vi "FiberMRI_Main_Protocol_NI.vi"() -> ()   [LabVIEW 2011]
doc: "Acquisition software for combined single-photon fluorescence and fMRI experiments."
uses:
  typedefs/storage_parameters_cluster.ctl
  typedefs/protocol_parameters.ctl
  typedefs/device_parameters.ctl
  typedefs/free_run_parameters.ctl
  typedefs/run_mode.ctl
  typedefs/main_state_enum.ctl
  typedefs/control_daq_enum.ctl
  typedefs/control_display_enum.ctl
  typedefs/control_storage_enum.ctl
  typedefs/control_analysis_enum.ctl
  <vilib>/Utility/error.llb/DialogType.ctl
  typedefs/control_shutter_enum.ctl
  typedefs/control_stim_enum.ctl
  typedefs/all_frontpanel_parameters_protocol_NI.ctl
  typedefs/experiment_mode_enum.ctl
  globals/exit.vi
panel:
  in  "Run mode":T1
  in  "Tab Control":T2(tab)
  in  "Protocol parameters":T3={"Repetitions"=1.0, "ON time"=40.0, "OFF time"=120.0, "Stim onset"=5.0, "Stim frequency"=1.0, "Pulse width"=1.0, "Acquire before ON"=1.0, "Acquire after ON"=1.0, "Sync shutter to acquisition"=TRUE} {"Pulse width" min=0.0001 max=0.1 step=0.01; "Acquire after ON" min=0.0 max=20.0 step=1.0; "Acquire before ON" min=0.0 max=20.0 step=1.0; "Repetitions" min=1.0 max=10.0 step=1.0; "OFF time" min=0.0 max=1000.0; "ON time" min=0.0 max=1000.0; "Stim onset" min=0.0 max=6000.0; "Stim frequency" min=-2.0 max=40.0 step=1.0}
  in  "Free run parameters":T4={"Stim onset"=5.0, "Stim frequency"=1.0, "Stim length"=0.001, "Sync shutter to acquisition"=TRUE} {"Stim length" min=0.0001 max=0.1 step=0.01; "Stim onset" min=0.0 max=100.0; "Stim frequency" min=0.1 max=40.0 step=1.0}
  in  "Storage parameters":T5
  in  "Device parameters":T6={"Triggered?"=FALSE, "Shutter channel"="", "Acquisition channels"="", "Acquisition sample rate"=100.0, "Read chunk size"=0, "Stimulation channel"="Dev1/ao0", "Stimulation sample rate"=100.0} {"Read chunk size" min=100 max=100000; "Acquisition sample rate" min=10.0 max=10000.0 step=10.0; "Stimulation sample rate" min=10.0 max=10000.0}
  out "Running":bool
  in  "Shutter":bool
  in  "Run":bool
  in  "Quit":bool
  # "Fiber - fMRI"
  # "_0000.txt"
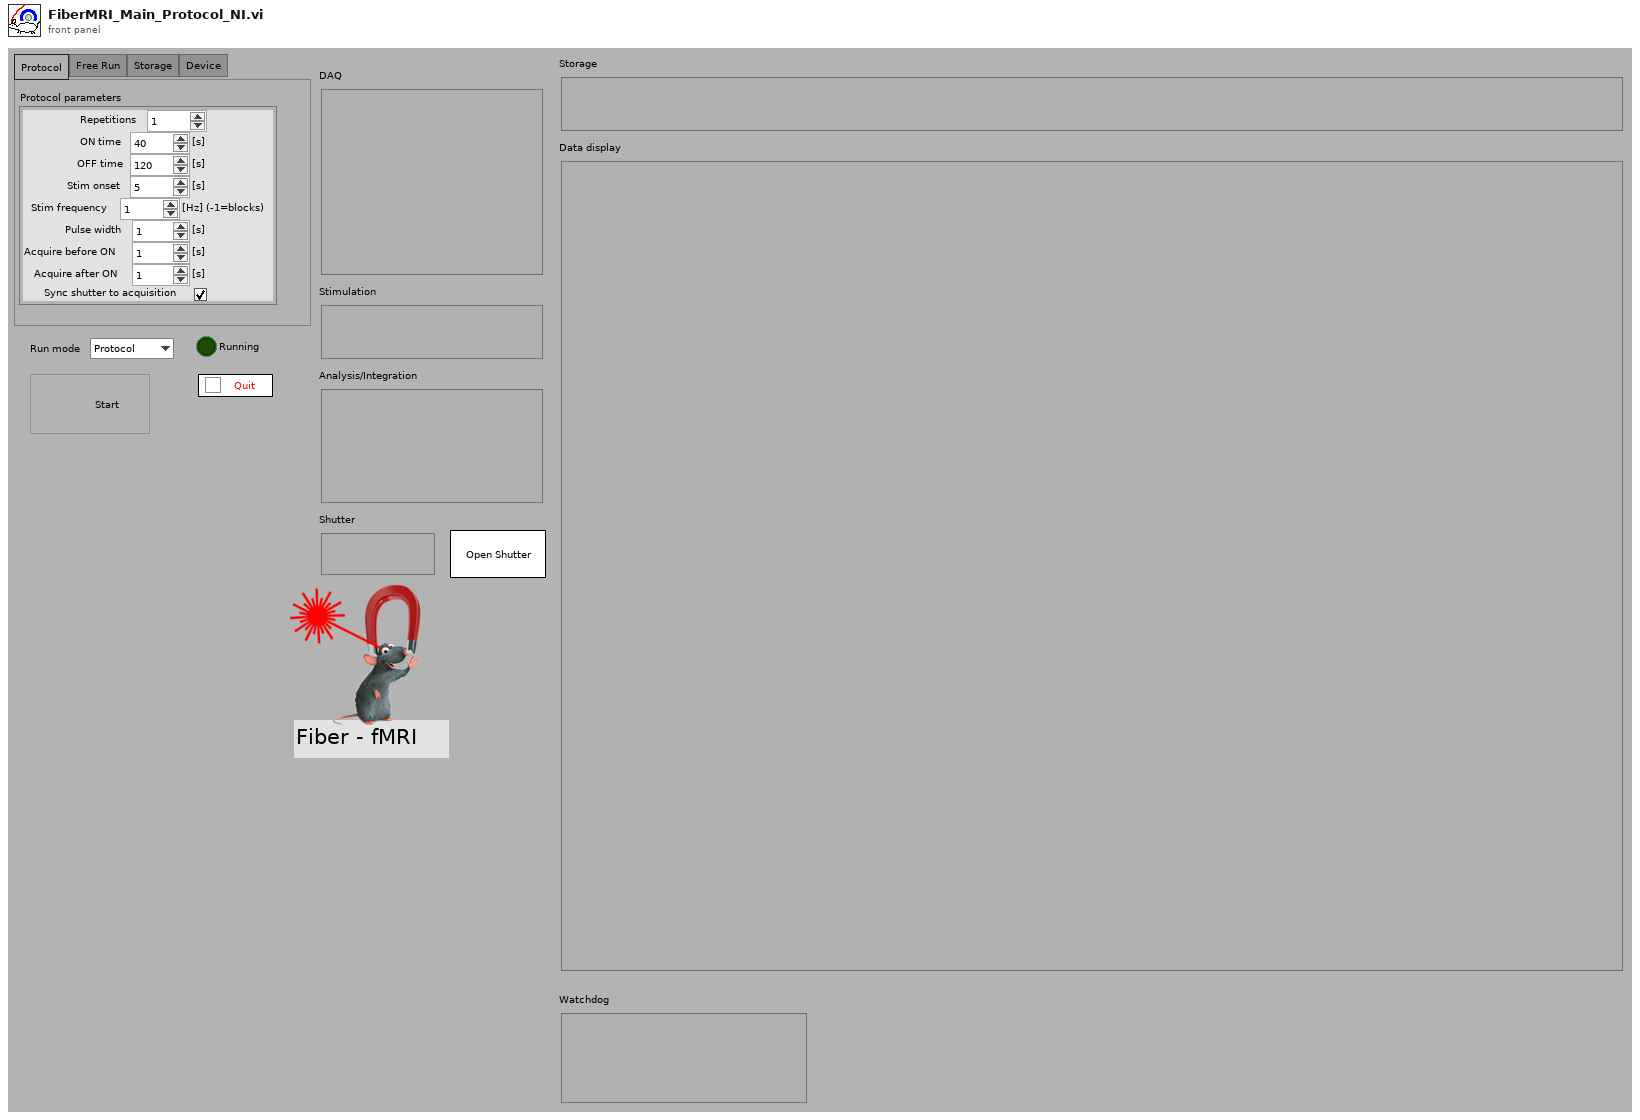
[diagram p1: front panel]
types:
  T1 = typedef "run_mode.ctl" = enum32{"Protocol", "Free Run"}
  T2 = enum32{"Protocol", "Free Run", "Storage", "Device"}
  T3 = typedef "protocol_parameters.ctl" = cluster{"Repetitions":dbl, "ON time":dbl, "OFF time":dbl, "Stim onset":dbl, "Stim frequency":dbl, "Pulse width":dbl, "Acquire before ON":dbl, "Acquire after ON":dbl, "Sync shutter to acquisition":bool}
  T4 = typedef "free_run_parameters.ctl" = cluster{"Stim onset":dbl, "Stim frequency":dbl, "Stim length":dbl, "Sync shutter to acquisition":bool}
  T5 = typedef "storage_parameters_cluster.ctl" = cluster{"Store?":bool, "Path":path, "Basename":string, "Auto-increment?":bool}
  T6 = typedef "device_parameters.ctl" = cluster{"Triggered?":bool, "Shutter channel":tag, "Acquisition channels":tag, "Acquisition sample rate":dbl, "Read chunk size":i32, "Stimulation channel":tag, "Stimulation sample rate":dbl}
  T7 = typedef "all_frontpanel_parameters_protocol_NI.ctl" = cluster{"Run mode":T1, "Protocol parameters":T3, "Free run parameters":T4, "Device parameters":T6, "Storage parameters":T5}
  T8 = typedef "DialogType.ctl" = u16
  T9 = typedef "main_state_enum.ctl" = enum16{"Init", "Empty", "ParamsChanged", "Start", "Stop", "Abort", "Acquisition finished", "SetShutter", "Reset", "Error", "Quit"}
  T10 = cluster{"Control_Stim_Queue":refnum<queue>, "Control_DAQ_Queue":refnum<queue>, "Control_Storage_Queue":refnum<queue>, "Control_Display_Queue":refnum<queue>, "Control_Analysis_Queue":refnum<queue>, "Control_Shutter_Queue":refnum<queue>}
  T11 = cluster{"Run mode":refnum<vi>, "Run":refnum<vi>, "Protocol parameters":refnum<vi>, "Tab Control":refnum<vi>, "Free run parameters":refnum<vi>, "Device parameters":refnum<vi>, "Storage parameters":refnum<vi>, "Shutter":refnum<vi>, "Quit":refnum<vi>}
  T12 = typedef "control_stim_enum.ctl" = enum16{"Init", "Stim Protocol", "Stim Free Run", "Stop", "Quit"}
  T13 = cluster{"Control stim Enum":T12, "variant":variant}
  T14 = typedef "control_shutter_enum.ctl" = enum16{"Init", "Open", "Close", "Quit"}
  T15 = cluster{"Control shutter enum":T14, "variant":variant}
  T16 = typedef "control_analysis_enum.ctl" = enum16{"Init", "Analyze", "Reset", "Stop", "Quit"}
  T17 = cluster{"Control Analysis Enum":T16, "variant":variant}
  T18 = typedef "control_display_enum.ctl" = enum16{"Init", "Display", "Quit"}
  T19 = cluster{"Control display enum":T18, "variant":variant}
  T20 = typedef "control_storage_enum.ctl" = enum16{"Init", "Discard", "Store", "Reset", "Stop", "Quit"}
  T21 = cluster{"Control storage enum":T20, "variant":variant}
  T22 = typedef "control_daq_enum.ctl" = enum16{"Init", "FreeRun", "Protocol", "Stop", "Quit"}
  T23 = cluster{"Control DAQ Enum":T22, "variant":variant}
  T24 = typedef "experiment_mode_enum.ctl" = enum32{"Raw data", "Measure background", "Measure F0", "Measure DF/F"}
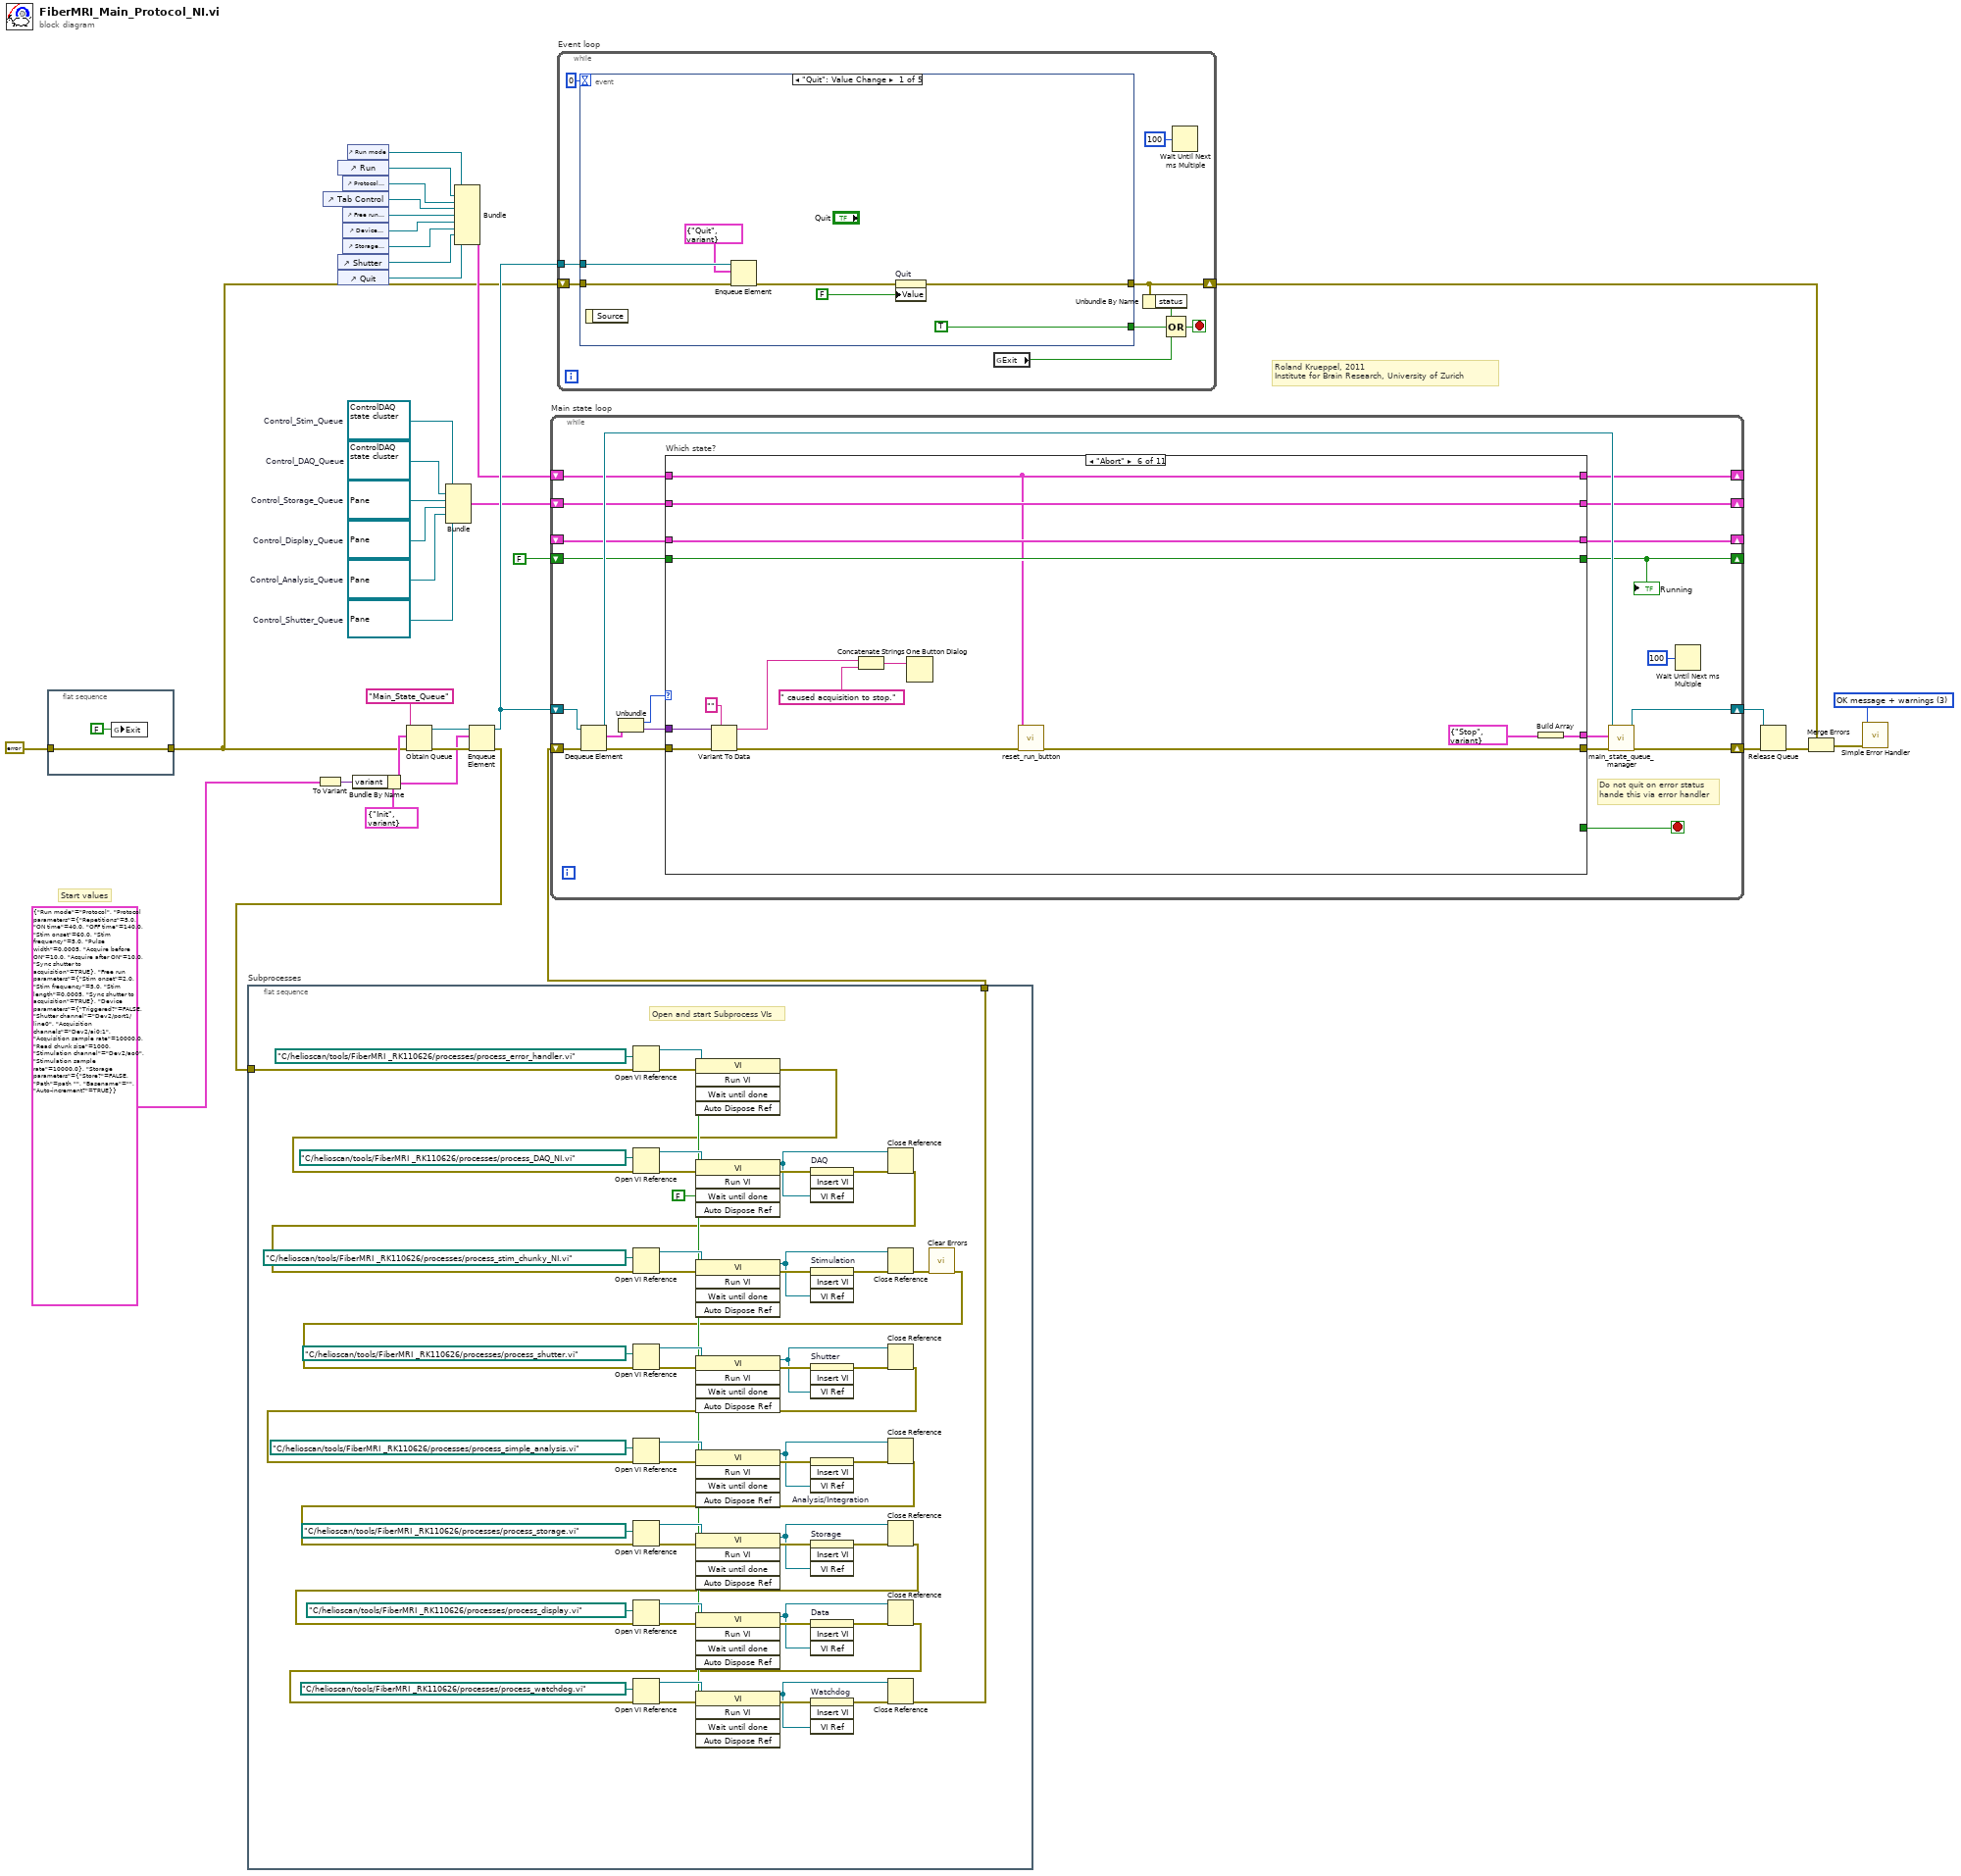
[diagram p0: block diagram]
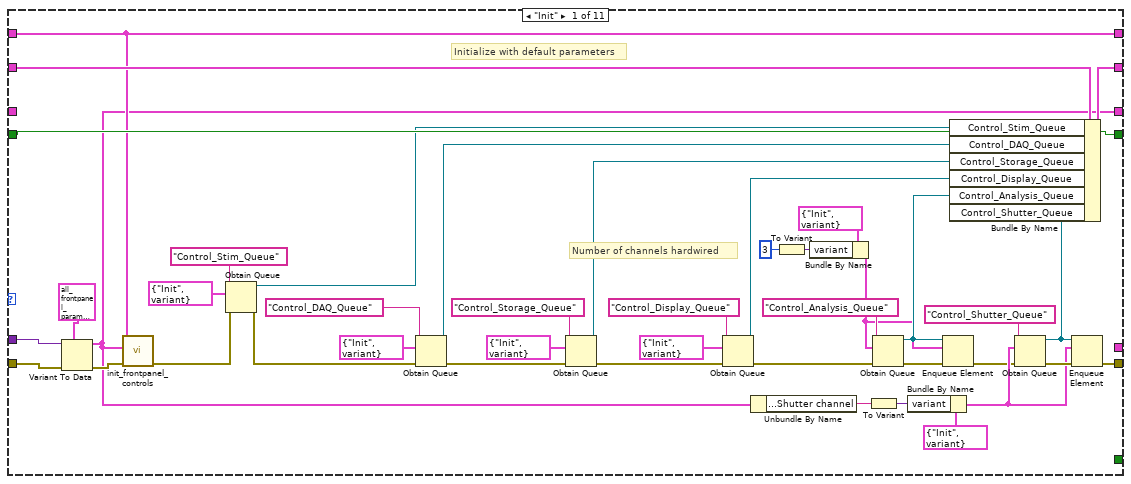
[diagram p2: hidden frame]
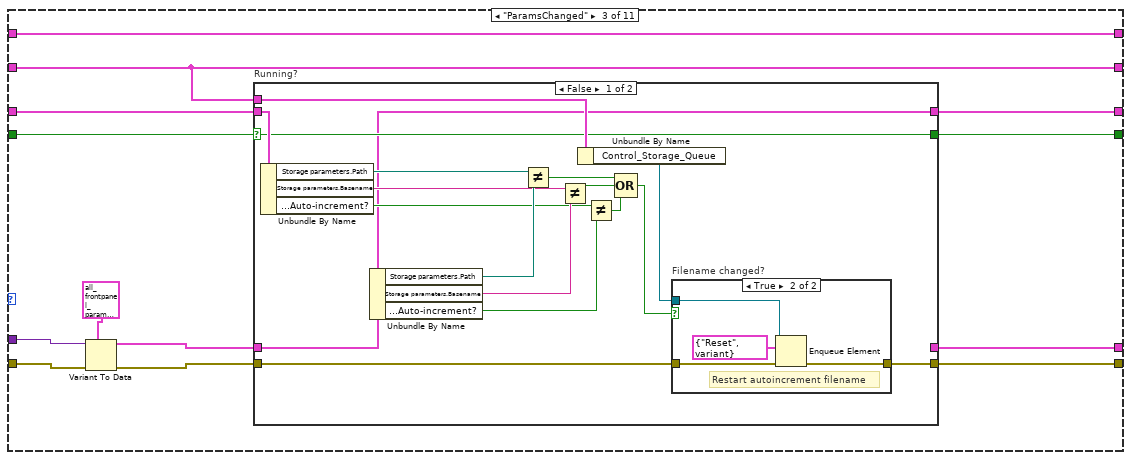
[diagram p4: hidden frame]
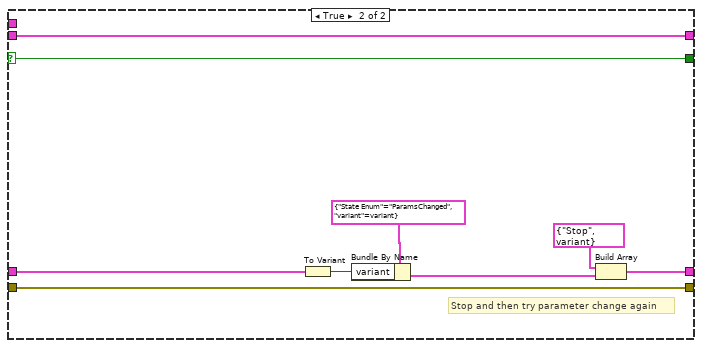
[diagram p6: hidden frame]
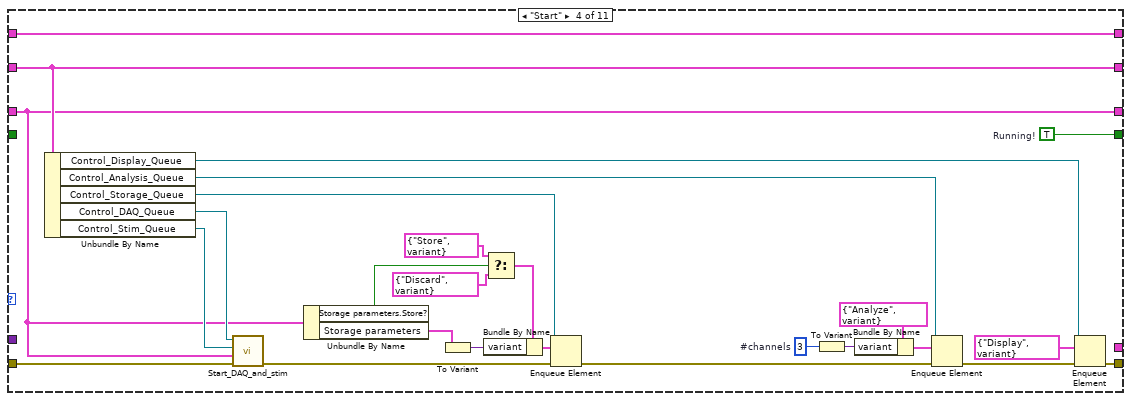
[diagram p7: hidden frame]
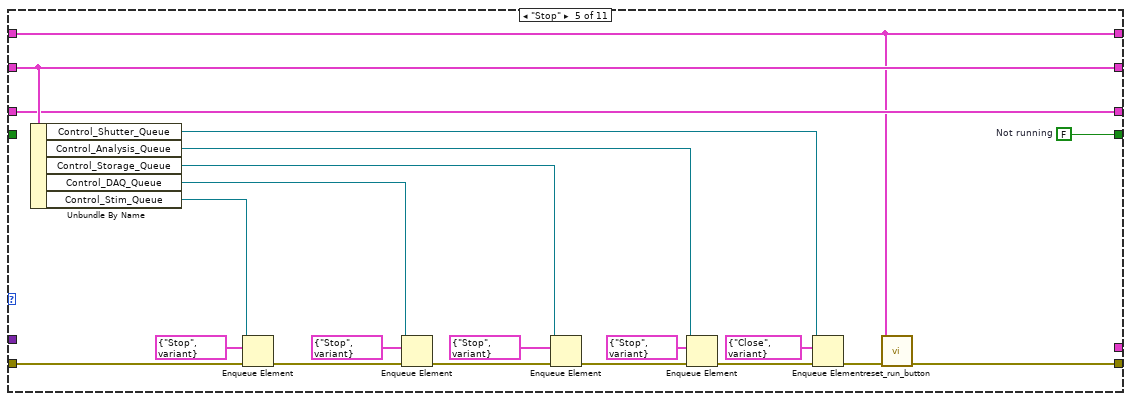
[diagram p8: hidden frame]
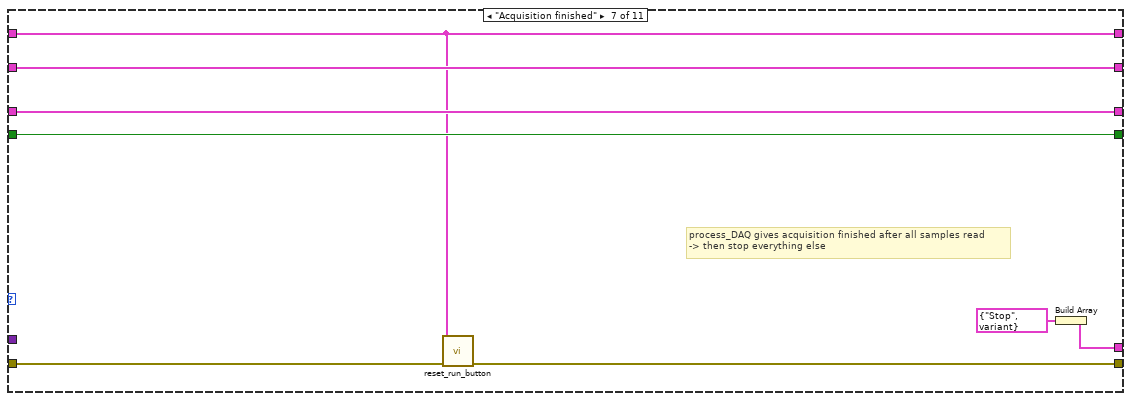
[diagram p9: hidden frame]
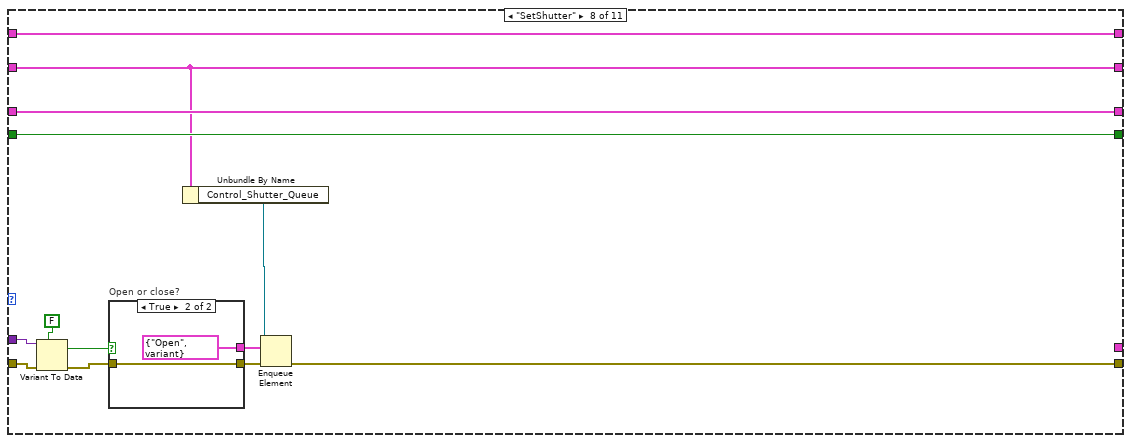
[diagram p10: hidden frame]
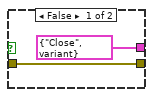
[diagram p11: hidden frame]
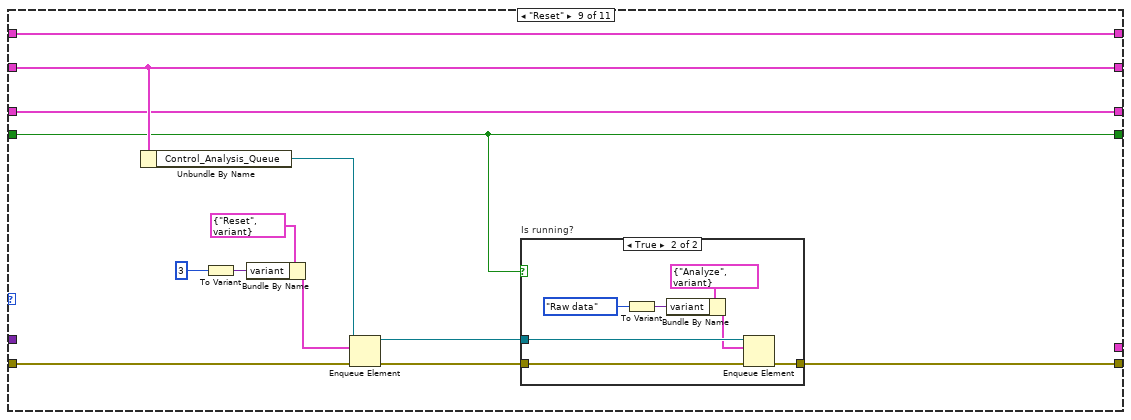
[diagram p12: hidden frame]
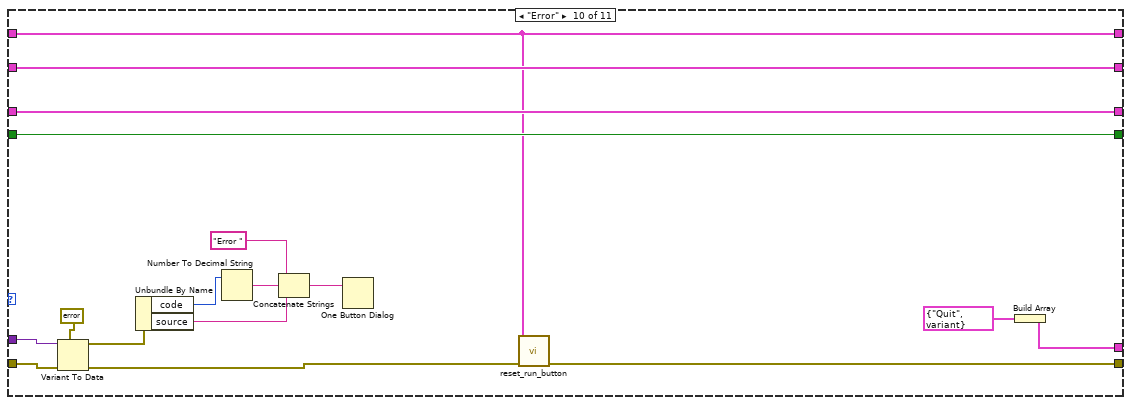
[diagram p14: hidden frame]
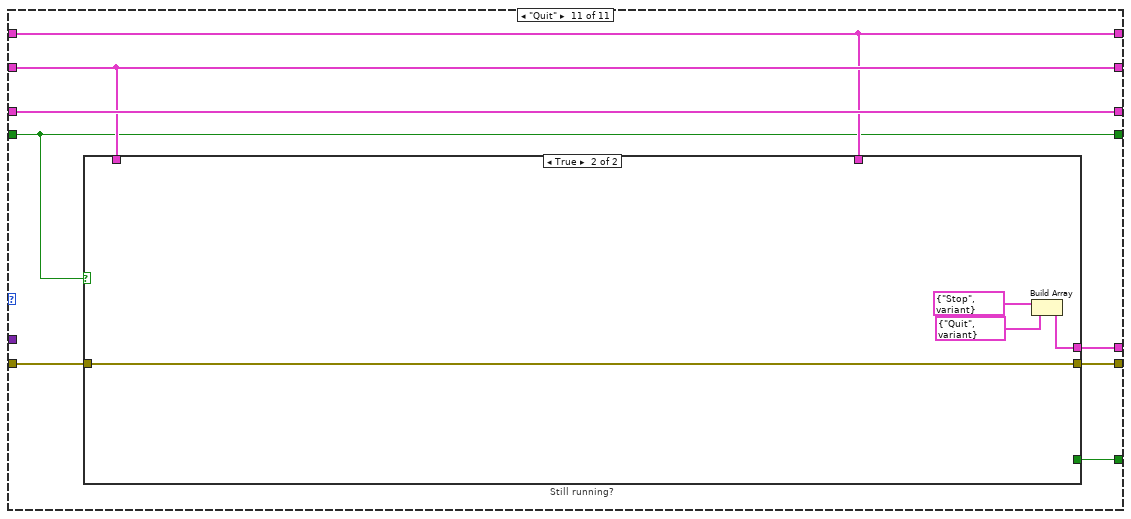
[diagram p15: hidden frame]
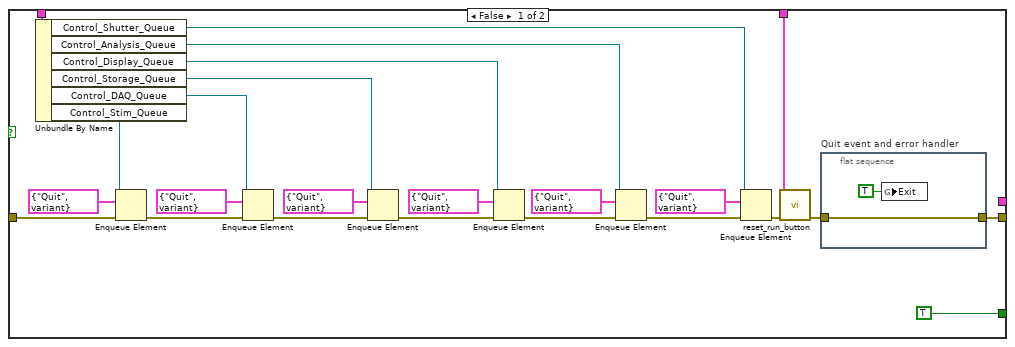
[diagram p16: hidden frame]
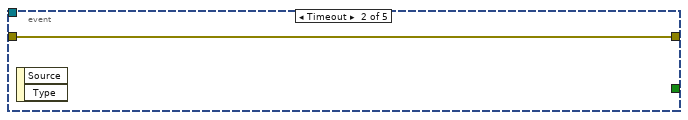
[diagram p17: hidden frame]
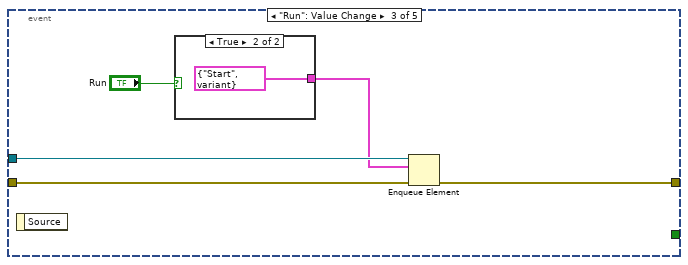
[diagram p18: hidden frame]
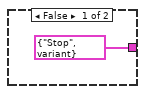
[diagram p19: hidden frame]
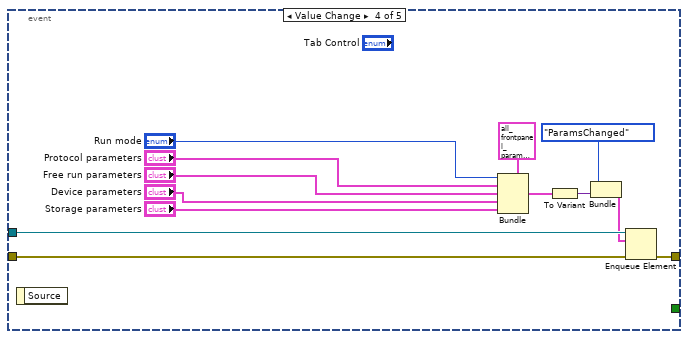
[diagram p20: hidden frame]
diagram:
  w16 = refnum<queue> refnum  # Control_Stim_Queue
  w17 = refnum<queue> refnum  # Control_Shutter_Queue
  w25 = T8 3 items=["no dialog", "OK message", "continue or stop message", "OK message + warnings", "continue/stop + warnings"] ("type of dialog (OK msg:1)")
  w26 = refnum<queue> refnum  # Control_Analysis_Queue
  w27 = refnum<queue> refnum  # Control_Storage_Queue
  w28 = refnum<queue> refnum  # Control_Display_Queue
  w30 = refnum<queue> refnum  # Control_DAQ_Queue
  # "Start values"
  # "Roland Krueppel, 2011\nInstitute for Brain Research, University of Zurich"
  n1 = flat-sequence {
    tunnel: errorcluster {"status"=FALSE, "code"=0, "source"=""} ("error out") -> [w37]
    tunnel: [w37] -> w3
    frame #0 {
      n2 = global write "exit.vi" "Exit"(FALSE ("Exit")) -> ()
    }
  }
  n3 = flat-sequence "Subprocesses" {
    tunnel: w2 -> [w43]
    tunnel: [w41] -> w1
    frame #0 {
      w49 = FALSE ("Wait Until Done")
      # "Open and start Subprocess VIs"
      n4 = Open VI Reference(vi path=path "C:/helioscan/tools/FiberMRI _RK110626/processes/process_error_handler.vi", error in (no error)=w43) -> (vi reference=w50:refnum<vi>, error out=w51:errorcluster)  [unwired: 4 in]
      n5 = invoke class="VI" method="Run VI"(reference=w50, error in=w51, "Wait until done"=w49) -> (error out=w42:errorcluster)  [unwired: 2 in, 4 out]
      n6 = Open VI Reference(vi path=path "C:/helioscan/tools/FiberMRI _RK110626/processes/process_DAQ_NI.vi", error in (no error)=w42) -> (vi reference=w89:refnum<vi>, error out=w90:errorcluster)  [unwired: 4 in]
      n7 = invoke class="VI" method="Run VI"(reference=w89, error in=w90, "Wait until done"=w49) -> (reference out=w68:refnum<vi>, error out=w70:errorcluster)  [unwired: 2 in, 3 out]
      n8 = invoke on="DAQ" class="SubPanel" method="Insert VI"(error in=w70, "VI Ref"=w68) -> (error out=w69:errorcluster)  [unwired: 2 in, 3 out]
      n9 = Close Reference(reference=w68, error in (no error)=w69) -> (error out=w48:errorcluster)
      n10 = Open VI Reference(vi path=path "C:/helioscan/tools/FiberMRI _RK110626/processes/process_stim_chunky_NI.vi", error in (no error)=w48) -> (vi reference=w58:refnum<vi>, error out=w59:errorcluster)  [unwired: 4 in]
      n11 = invoke class="VI" method="Run VI"(reference=w58, error in=w59, "Wait until done"=w49) -> (reference out=w54:refnum<vi>, error out=w56:errorcluster)  [unwired: 2 in, 3 out]
      n12 = invoke on="Stimulation" class="SubPanel" method="Insert VI"(error in=w56, "VI Ref"=w54) -> (error out=w55:errorcluster)  [unwired: 2 in, 3 out]
      n13 = Close Reference(reference=w54, error in (no error)=w55) -> (error out=w40:errorcluster)
      n14 = call <vilib>:"Clear Errors.vi"("error in (no error)"=w40) -> ("error out"=w39:errorcluster)  [unwired: 6 in]
      n15 = Open VI Reference(vi path=path "C:/helioscan/tools/FiberMRI _RK110626/processes/process_shutter.vi", error in (no error)=w39) -> (vi reference=w53:refnum<vi>, error out=w63:errorcluster)  [unwired: 4 in]
      n16 = invoke class="VI" method="Run VI"(reference=w53, error in=w63, "Wait until done"=w49) -> (reference out=w60:refnum<vi>, error out=w62:errorcluster)  [unwired: 2 in, 3 out]
      n17 = invoke on="Shutter" class="SubPanel" method="Insert VI"(error in=w62, "VI Ref"=w60) -> (error out=w61:errorcluster)  [unwired: 2 in, 3 out]
      n18 = Close Reference(reference=w60, error in (no error)=w61) -> (error out=w47:errorcluster)
      n19 = Open VI Reference(vi path=path "C:/helioscan/tools/FiberMRI _RK110626/processes/process_simple_analysis.vi", error in (no error)=w47) -> (vi reference=w87:refnum<vi>, error out=w88:errorcluster)  [unwired: 4 in]
      n20 = invoke class="VI" method="Run VI"(reference=w87, error in=w88, "Wait until done"=w49) -> (reference out=w79:refnum<vi>, error out=w82:errorcluster)  [unwired: 2 in, 3 out]
      n21 = invoke on="Analysis/Integration" class="SubPanel" method="Insert VI"(error in=w82, "VI Ref"=w79) -> (error out=w80:errorcluster)  [unwired: 2 in, 3 out]
      n22 = Close Reference(reference=w79, error in (no error)=w80) -> (error out=w46:errorcluster)
      n23 = Open VI Reference(vi path=path "C:/helioscan/tools/FiberMRI _RK110626/processes/process_storage.vi", error in (no error)=w46) -> (vi reference=w85:refnum<vi>, error out=w86:errorcluster)  [unwired: 4 in]
      n24 = invoke class="VI" method="Run VI"(reference=w85, error in=w86, "Wait until done"=w49) -> (reference out=w65:refnum<vi>, error out=w67:errorcluster)  [unwired: 2 in, 3 out]
      n25 = invoke on="Storage" class="SubPanel" method="Insert VI"(error in=w67, "VI Ref"=w65) -> (error out=w66:errorcluster)  [unwired: 2 in, 3 out]
      n26 = Close Reference(reference=w65, error in (no error)=w66) -> (error out=w45:errorcluster)
      n27 = Open VI Reference(vi path=path "C:/helioscan/tools/FiberMRI _RK110626/processes/process_display.vi", error in (no error)=w45) -> (vi reference=w83:refnum<vi>, error out=w84:errorcluster)  [unwired: 4 in]
      n28 = invoke class="VI" method="Run VI"(reference=w83, error in=w84, "Wait until done"=w49) -> (reference out=w77:refnum<vi>, error out=w81:errorcluster)  [unwired: 2 in, 3 out]
      n29 = invoke on="Data" class="SubPanel" method="Insert VI"(error in=w81, "VI Ref"=w77) -> (error out=w78:errorcluster)  [unwired: 2 in, 3 out]
      n30 = Close Reference(reference=w77, error in (no error)=w78) -> (error out=w44:errorcluster)
      n31 = Open VI Reference(vi path=path "C:/helioscan/tools/FiberMRI _RK110626/processes/process_watchdog.vi", error in (no error)=w44) -> (vi reference=w74:refnum<vi>, error out=w76:errorcluster)  [unwired: 4 in]
      n32 = invoke class="VI" method="Run VI"(reference=w74, error in=w76, "Wait until done"=w49) -> (reference out=w71:refnum<vi>, error out=w73:errorcluster)  [unwired: 2 in, 3 out]
      n33 = invoke on="Watchdog" class="SubPanel" method="Insert VI"(error in=w73, "VI Ref"=w71) -> (error out=w72:errorcluster)  [unwired: 2 in, 3 out]
      n34 = Close Reference(reference=w71, error in (no error)=w72) -> (error out=w41:errorcluster)
    }
  }
  n35 = To Variant(anything=T7 {"Run mode"=enum."Protocol", "Protocol parameters"={"Repetitions"=5.0, "ON time"=40.0, "OFF time"=140.0, "Stim onset"=60.0, "Stim frequency"=5.0, "Pulse width"=0.0005, "Acquire before ON"=10.0, "Acquire after ON"=10.0, "Sync shutter to acquisition"=TRUE}, "Free run parameters"={"Stim onset"=2.0, "Stim frequency"=5.0, "Stim length"=0.0005, "Sync shutter to acquisition"=TRUE}, "Device parameters"={"Triggered?"=FALSE, "Shutter channel"="Dev2/port1/line0", "Acquisition channels"="Dev2/ai0:1", "Acquisition sample rate"=10000.0, "Read chunk size"=1000, "Stimulation channel"="Dev2/ao0", "Stimulation sample rate"=10000.0}, "Storage parameters"={"Store?"=FALSE, "Path"=path "", "Basename"="", "Auto-increment?"=TRUE}} ("All frontpanel parameters")) -> (Variant=w19:variant)
  n36 = control-ref of="Tab Control"() -> (w12:refnum<vi>)
  n37 = control-ref of="Run"() -> (w14:refnum<vi>)
  n38 = control-ref of="Shutter"() -> (w8:refnum<vi>)
  n39 = control-ref of="Quit"() -> (w7:refnum<vi>)
  n40 = control-ref of="Protocol parameters"() -> (w13:refnum<vi>)
  n41 = control-ref of="Free run parameters"() -> (w11:refnum<vi>)
  n42 = control-ref of="Device parameters"() -> (w10:refnum<vi>)
  n43 = control-ref of="Storage parameters"() -> (w9:refnum<vi>)
  n44 = control-ref of="Run mode"() -> (w15:refnum<vi>)
  n45 = Bundle By Name(cluster=cluster{"State Enum":T9, "variant":variant} {"State Enum"=enum."Init", "variant"=variant}, "variant"=w19) -> (w18:cluster{"State Enum":T9, "variant":variant})
  n46 = Obtain Queue(name (unnamed)="Main_State_Queue", element data type=w18, error in (no error)=w3) -> (queue out=w35:refnum<queue>, error out=w33:errorcluster)  [unwired: 2 in, 1 out]
  n47 = Bundle("Control_Stim_Queue"=w16, "Control_DAQ_Queue"=w30, "Control_Storage_Queue"=w27, "Control_Display_Queue"=w28, "Control_Analysis_Queue"=w26, "Control_Shutter_Queue"=w17) -> (w29:T10)  [unwired: 1 in]
  n48 = Bundle("Run mode"=w15, "Run"=w14, "Protocol parameters"=w13, "Tab Control"=w12, "Free run parameters"=w11, "Device parameters"=w10, "Storage parameters"=w9, "Shutter"=w8, "Quit"=w7) -> (w6:T11)  [unwired: 1 in]
  n49 = Enqueue Element(queue=w35, element=w18, error in (no error)=w33) -> (queue out=w34:refnum<queue>, error out=w2:errorcluster)  [unwired: 1 in, 1 out]
  n50 = while "Main state loop" {
    shift-right: [w96] -> w36
    shift-left: w1 -> [w113]
    shift-right: [w108] -> _
    shift-left: _ -> [w107]
    shift-right: [w105] -> _
    shift-left: w29 -> [w106]
    shift-right: [w103] -> _
    shift-left: FALSE -> [w104]
    shift-right: [w97] -> _
    shift-left: w6 -> [w98]
    shift-right: [w99] -> w32
    shift-left: w34 -> [w114]
    stop <- w95 stop-if-true
    # "Do not quit on error status\nhande this via error handler"
    n51 = Dequeue Element(queue=w114, error in (no error)=w113) -> (queue out=w115:refnum<queue>, element=w111:cluster{"State Enum":T9, "variant":variant}, error out=w112:errorcluster)  [unwired: 1 in, 1 out]
    n52 = Unbundle(w111) -> ("State Enum"=w110:T9, "variant"=w109:variant)
    n53 = case "Which state?" shown="\"Abort\"" w110 {
      tunnel: w112 -> [w141 w162 w174 w214 w242 w264 w270 w287 w304 w324 w336]
      tunnel: [w132 w162 w170 w230 w234 w255 w269 w277 w300 w327 w334] -> w101
      tunnel: w109 -> [w140 _ w175 _ _ w263 _ w286 _ w325 _]
      tunnel: [w116 w161 w165 w209 w244 w267 w275 w288 w302 w330 w338] -> w108
      tunnel: w107 -> [_ w161 w173 w209 w244 w267 w275 w288 w302 w330 w338]
      tunnel: w106 -> [w153 w160 w172 w232 w252 w266 w274 w283 w305 w329 w337]
      tunnel: [w152 w160 w172 w232 w252 w266 w274 w283 w305 w329 w337] -> w105
      tunnel: w104 -> [w142 w159 w168 _ _ w265 w271 w284 w298 w328 w333]
      tunnel: [w142 w159 w167 w221 w243 w265 w271 w284 w298 w328 w333] -> w103
      tunnel: [_ _ w164 _ _ w257 w272 _ _ w314 w332] -> w100
      tunnel: w98 -> [w117 w158 w163 w207 w233 w254 w268 w276 w293 w326 w335]
      tunnel: [w117 w158 w163 w207 w233 w254 w268 w276 w293 w326 w335] -> w97
      tunnel: [_ _ _ _ _ _ _ _ _ _ w331] -> w95
      frame "Init" {
        # "Number of channels hardwired"
        # "Initialize with default parameters"
        n54 = Variant To Data(error in=w141, type=T7 {"Run mode"=enum."Protocol", "Protocol parameters"={"Repetitions"=0.0, "ON time"=0.0, "OFF time"=0.0, "Stim onset"=0.0, "Stim frequency"=0.0, "Pulse width"=0.0, "Acquire before ON"=0.0, "Acquire after ON"=0.0, "Sync shutter to acquisition"=FALSE}, "Free run parameters"={"Stim onset"=0.0, "Stim frequency"=0.0, "Stim length"=0.0, "Sync shutter to acquisition"=FALSE}, "Device parameters"={"Triggered?"=FALSE, "Shutter channel"="", "Acquisition channels"="", "Acquisition sample rate"=0.0, "Read chunk size"=0, "Stimulation channel"="", "Stimulation sample rate"=0.0}, "Storage parameters"={"Store?"=FALSE, "Path"=path "", "Basename"="", "Auto-increment?"=FALSE}} ("All frontpanel parameters"), Variant=w140) -> (data=w116:T7, error out=w119:errorcluster)
        n55 = call "init_frontpanel_controls.vi"("error in"=w119, "All frontpanel parameters"=w116, "All frontpanel references"=w117) -> ("error out"=w118:errorcluster)  [unwired: 8 in]
        n56 = Obtain Queue(name (unnamed)="Control_Stim_Queue", element data type=T13 {"Control stim Enum"=enum."Init", "variant"=variant} ("ControlDAQ state cluster"), error in (no error)=w118) -> (queue out=w130:refnum<queue>, error out=w120:errorcluster)  [unwired: 2 in, 1 out]
        n57 = Obtain Queue(name (unnamed)="Control_DAQ_Queue", element data type=T23 {"Control DAQ Enum"=enum."Init", "variant"=variant} ("ControlDAQ state cluster"), error in (no error)=w120) -> (queue out=w151:refnum<queue>, error out=w149:errorcluster)  [unwired: 2 in, 1 out]
        n58 = Obtain Queue(name (unnamed)="Control_Storage_Queue", element data type=T21 {"Control storage enum"=enum."Init", "variant"=variant}, error in (no error)=w149) -> (queue out=w150:refnum<queue>, error out=w148:errorcluster)  [unwired: 2 in, 1 out]
        n59 = Obtain Queue(name (unnamed)="Control_Display_Queue", element data type=T19 {"Control display enum"=enum."Init", "variant"=variant}, error in (no error)=w148) -> (queue out=w145:refnum<queue>, error out=w144:errorcluster)  [unwired: 2 in, 1 out]
        n60 = Unbundle By Name(w116) -> ("Device parameters.Shutter channel"=w137:tag)
        n61 = To Variant(anything=3) -> (Variant=w125:variant)
        n62 = Bundle By Name(cluster=T17 {"Control Analysis Enum"=enum."Init", "variant"=variant}, "variant"=w125) -> (w121:T17)
        n63 = To Variant(anything=w137) -> (Variant=w135:variant)
        n64 = Obtain Queue(name (unnamed)="Control_Analysis_Queue", element data type=w121, error in (no error)=w144) -> (queue out=w122:refnum<queue>, error out=w124:errorcluster)  [unwired: 2 in, 1 out]
        n65 = Bundle By Name(cluster=T15 {"Control shutter enum"=enum."Init", "variant"=variant}, "variant"=w135) -> (w131:T15)
        n66 = Enqueue Element(queue=w122, element=w121, error in (no error)=w124) -> (error out=w123:errorcluster)  [unwired: 1 in, 2 out]
        n67 = Obtain Queue(name (unnamed)="Control_Shutter_Queue", element data type=w131, error in (no error)=w123) -> (queue out=w134:refnum<queue>, error out=w133:errorcluster)  [unwired: 2 in, 1 out]
        n68 = Bundle By Name(cluster=w153, "Control_Stim_Queue"=w130, "Control_DAQ_Queue"=w151, "Control_Storage_Queue"=w150, "Control_Display_Queue"=w145, "Control_Analysis_Queue"=w122, "Control_Shutter_Queue"=w134) -> (w152:T10)
        n69 = Enqueue Element(queue=w134, element=w131, error in (no error)=w133) -> (error out=w132:errorcluster)  [unwired: 1 in, 2 out]
      }
      frame "Empty", Default {
        # "Do nothing"
      }
      frame "ParamsChanged" {
        n70 = Variant To Data(error in=w174, type=T7 {"Run mode"=enum."Protocol", "Protocol parameters"={"Repetitions"=0.0, "ON time"=0.0, "OFF time"=0.0, "Stim onset"=0.0, "Stim frequency"=0.0, "Pulse width"=0.0, "Acquire before ON"=0.0, "Acquire after ON"=0.0, "Sync shutter to acquisition"=FALSE}, "Free run parameters"={"Stim onset"=0.0, "Stim frequency"=0.0, "Stim length"=0.0, "Sync shutter to acquisition"=FALSE}, "Device parameters"={"Triggered?"=FALSE, "Shutter channel"="", "Acquisition channels"="", "Acquisition sample rate"=0.0, "Read chunk size"=0, "Stimulation channel"="", "Stimulation sample rate"=0.0}, "Storage parameters"={"Store?"=FALSE, "Path"=path "", "Basename"="", "Auto-increment?"=FALSE}} ("All frontpanel parameters"), Variant=w175) -> (data=w166:T7, error out=w171:errorcluster)
        n71 = case "Running?" shown="False" w168 {
          selector: w168 -> [w177 w206]
          tunnel: w173 -> [w192 w199]
          tunnel: w172 -> [w181 _]
          tunnel: w171 -> [w179 w198]
          tunnel: [w178 w198] -> w170
          tunnel: w166 -> [w176 w205]
          tunnel: [w177 w206] -> w167
          tunnel: [w176 w199] -> w165
          tunnel: [_ w201] -> w164
          frame False {
            n72 = Unbundle By Name(w192) -> ("Storage parameters.Path"=w191:path, "Storage parameters.Basename"=w189:string, "Storage parameters.Auto-increment?"=w187:bool)
            n73 = Unbundle By Name(w176) -> ("Storage parameters.Path"=w190:path, "Storage parameters.Basename"=w188:string, "Storage parameters.Auto-increment?"=w186:bool)
            n74 = Not Equal?(x=w191, y=w190) -> (x != y?=w185:bool)
            n75 = Not Equal?(x=w189, y=w188) -> (x != y?=w184:bool)
            n76 = Unbundle By Name(w181) -> ("Control_Storage_Queue"=w180:refnum<queue>)
            n77 = Not Equal?(x=w187, y=w186) -> (x != y?=w183:bool)
            n78 = Compound Arithmetic op=OR(w185, w184, w183) -> (w182:bool)
            n79 = case "Filename changed?" shown="True" w182 {
              tunnel: w180 -> [_ w197]
              tunnel: w179 -> [w193 w195]
              tunnel: [w193 w194] -> w178
              frame False {
              }
              frame True {
                # "Restart autoincrement filename"
                n80 = Enqueue Element(queue=w197, element=T21 {"Control storage enum"=enum."Reset", "variant"=variant}, error in (no error)=w195) -> (error out=w194:errorcluster)  [unwired: 1 in, 2 out]
              }
            }
          }
          frame True {
            # "Stop and then try parameter change again"
            n81 = To Variant(anything=w205) -> (Variant=w203:variant)
            n82 = Bundle By Name(cluster=cluster{"State Enum":T9, "variant":variant} {"State Enum"=enum."ParamsChanged", "variant"=variant}, "variant"=w203) -> (w200:cluster{"State Enum":T9, "variant":variant})
            n83 = Build Array(cluster{"State Enum":T9, "variant":variant} {"State Enum"=enum."Stop", "variant"=variant}, w200) -> (w201:cluster{"State Enum":T9, "variant":variant}[])
          }
        }
      }
      frame "Start" {
        w208 = 3  # #channels
        w221 = TRUE  # Running!
        n84 = Unbundle By Name(w232) -> ("Control_Display_Queue"=w228:refnum<queue>, "Control_Analysis_Queue"=w225:refnum<queue>, "Control_Storage_Queue"=w231:refnum<queue>, "Control_DAQ_Queue"=w212:refnum<queue>, "Control_Stim_Queue"=w211:refnum<queue>)
        n85 = call "Start_DAQ_and_stim.vi"("error in"=w214, "All frontpanel parameters"=w209, "Control_Stim_Queue"=w211, "Control_DAQ_Queue"=w212) -> ("error out"=w213:errorcluster)  [unwired: 5 in]
        n86 = Unbundle By Name(w209) -> ("Storage parameters.Store?"=w210:bool, "Storage parameters"=w220:T5)
        n87 = To Variant(anything=w220) -> (Variant=w219:variant)
        n88 = Select(t=T21 {"Control storage enum"=enum."Store", "variant"=variant} ("element"), s=w210, f=T21 {"Control storage enum"=enum."Discard", "variant"=variant} ("element")) -> (s? t:f=w216:T21)
        n89 = Bundle By Name(cluster=w216, "variant"=w219) -> (w215:T21)
        n90 = Enqueue Element(queue=w231, element=w215, error in (no error)=w213) -> (error out=w227:errorcluster)  [unwired: 1 in, 2 out]
        n91 = To Variant(anything=w208) -> (Variant=w224:variant)
        n92 = Bundle By Name(cluster=T17 {"Control Analysis Enum"=enum."Analyze", "variant"=variant} ("element"), "variant"=w224) -> (w222:T17)
        n93 = Enqueue Element(queue=w225, element=w222, error in (no error)=w227) -> (error out=w226:errorcluster)  [unwired: 1 in, 2 out]
        n94 = Enqueue Element(queue=w228, element=T19 {"Control display enum"=enum."Display", "variant"=variant}, error in (no error)=w226) -> (error out=w230:errorcluster)  [unwired: 1 in, 2 out]
      }
      frame "Stop" {
        w243 = FALSE  # Not running
        n95 = Unbundle By Name(w252) -> ("Control_Shutter_Queue"=w237:refnum<queue>, "Control_Analysis_Queue"=w246:refnum<queue>, "Control_Storage_Queue"=w249:refnum<queue>, "Control_DAQ_Queue"=w251:refnum<queue>, "Control_Stim_Queue"=w240:refnum<queue>)
        n96 = Enqueue Element(queue=w240, element=T13 {"Control stim Enum"=enum."Stop", "variant"=variant}, error in (no error)=w242) -> (error out=w241:errorcluster)  [unwired: 1 in, 2 out]
        n97 = Enqueue Element(queue=w251, element=T23 {"Control DAQ Enum"=enum."Stop", "variant"=variant}, error in (no error)=w241) -> (error out=w250:errorcluster)  [unwired: 1 in, 2 out]
        n98 = Enqueue Element(queue=w249, element=T21 {"Control storage enum"=enum."Stop", "variant"=variant}, error in (no error)=w250) -> (error out=w247:errorcluster)  [unwired: 1 in, 2 out]
        n99 = Enqueue Element(queue=w246, element=T17 {"Control Analysis Enum"=enum."Stop", "variant"=variant}, error in (no error)=w247) -> (error out=w238:errorcluster)  [unwired: 1 in, 2 out]
        n100 = Enqueue Element(queue=w237, element=T15 {"Control shutter enum"=enum."Close", "variant"=variant}, error in (no error)=w238) -> (error out=w235:errorcluster)  [unwired: 1 in, 2 out]
        n101 = call "reset_run_button.vi"("error in"=w235, "Front panel references"=w233) -> ("error out"=w234:errorcluster)  [unwired: 7 in]
      }
      frame "Abort" {
        n102 = Variant To Data(error in=w264, type="", Variant=w263) -> (data=w261:string, error out=w256:errorcluster)
        n103 = Concatenate Strings(w261, " caused acquisition to stop.") -> (w259:string)
        n104 = One Button Dialog(message=w259) -> ()  [unwired: 1 in, 1 out]
        n105 = call "reset_run_button.vi"("error in"=w256, "Front panel references"=w254) -> ("error out"=w255:errorcluster)  [unwired: 7 in]
        n106 = Build Array(cluster{"State Enum":T9, "variant":variant} {"State Enum"=enum."Stop", "variant"=variant}) -> (w257:cluster{"State Enum":T9, "variant":variant}[])
      }
      frame "Acquisition finished" {
        # "process_DAQ gives acquisition finished after all samples read\n-> then stop everything else"
        n107 = call "reset_run_button.vi"("error in"=w270, "Front panel references"=w268) -> ("error out"=w269:errorcluster)  [unwired: 7 in]
        n108 = Build Array(cluster{"State Enum":T9, "variant":variant} {"State Enum"=enum."Stop", "variant"=variant}) -> (w272:cluster{"State Enum":T9, "variant":variant}[])
      }
      frame "SetShutter" {
        n109 = Variant To Data(error in=w287, type=FALSE, Variant=w286) -> (data=w281:bool, error out=w280:errorcluster)
        n110 = case "Open or close?" shown="True" w281 {
          tunnel: [w290 w292] -> w279
          tunnel: w280 -> [w290 w292]
          tunnel: [T15 {"Control shutter enum"=enum."Close", "variant"=variant} ("element") T15 {"Control shutter enum"=enum."Open", "variant"=variant} ("element")] -> w278
          frame False {
          }
          frame True {
          }
        }
        n111 = Unbundle By Name(w283) -> ("Control_Shutter_Queue"=w282:refnum<queue>)
        n112 = Enqueue Element(queue=w282, element=w278, error in (no error)=w279) -> (error out=w277:errorcluster)  [unwired: 1 in, 2 out]
      }
      frame "Reset" {
        n113 = Unbundle By Name(w305) -> ("Control_Analysis_Queue"=w303:refnum<queue>)
        n114 = To Variant(anything=3) -> (Variant=w295:variant)
        n115 = Bundle By Name(cluster=T17 {"Control Analysis Enum"=enum."Reset", "variant"=variant} ("element"), "variant"=w295) -> (w294:T17)
        n116 = Enqueue Element(queue=w303, element=w294, error in (no error)=w304) -> (queue out=w299:refnum<queue>, error out=w301:errorcluster)  [unwired: 1 in, 1 out]
        n117 = case "Is running?" shown="True" w298 {
          tunnel: [w306 w312] -> w300
          tunnel: w301 -> [w306 w313]
          tunnel: w299 -> [_ w311]
          frame False {
          }
          frame True {
            n118 = To Variant(anything=experiment_mode_enum."Raw data" ("Experiment mode")) -> (Variant=w308:variant)
            n119 = Bundle By Name(cluster=T17 {"Control Analysis Enum"=enum."Analyze", "variant"=variant} ("element"), "variant"=w308) -> (w309:T17)
            n120 = Enqueue Element(queue=w311, element=w309, error in (no error)=w313) -> (error out=w312:errorcluster)  [unwired: 1 in, 2 out]
          }
        }
      }
      frame "Error" {
        n121 = Variant To Data(error in=w324, type=errorcluster {"status"=FALSE, "code"=0, "source"=""} ("error IO"), Variant=w325) -> (data=w321:errorcluster, error out=w323:errorcluster)
        n122 = Unbundle By Name(w321) -> ("code"=w320:i32, "source"=w317:string)
        n123 = Number To Decimal String(number=w320) -> (decimal integer string=w318:string)  [unwired: 1 in]
        n124 = Concatenate Strings("Error ", w318, w317) -> (w316:string)
        n125 = One Button Dialog(message=w316) -> ()  [unwired: 1 in, 1 out]
        n126 = call "reset_run_button.vi"("error in"=w323, "Front panel references"=w326) -> ("error out"=w327:errorcluster)  [unwired: 7 in]
        n127 = Build Array(cluster{"State Enum":T9, "variant":variant} {"State Enum"=enum."Quit", "variant"=variant} ("element")) -> (w314:cluster{"State Enum":T9, "variant":variant}[])
      }
      frame "Quit" {
        n128 = case "Still running?" shown="True" w333 {
          tunnel: w337 -> [w361 _]
          tunnel: w336 -> [w350 w365]
          tunnel: w335 -> [w342 _]
          tunnel: [w340 w365] -> w334
          tunnel: [_ w366] -> w332
          tunnel: [TRUE _] -> w331
          frame False {
            n129 = Unbundle By Name(w361) -> ("Control_Shutter_Queue"=w345:refnum<queue>, "Control_Analysis_Queue"=w352:refnum<queue>, "Control_Display_Queue"=w355:refnum<queue>, "Control_Storage_Queue"=w358:refnum<queue>, "Control_DAQ_Queue"=w360:refnum<queue>, "Control_Stim_Queue"=w348:refnum<queue>)
            n130 = Enqueue Element(queue=w348, element=T13 {"Control stim Enum"=enum."Quit", "variant"=variant}, error in (no error)=w350) -> (error out=w349:errorcluster)  [unwired: 1 in, 2 out]
            n131 = Enqueue Element(queue=w360, element=T23 {"Control DAQ Enum"=enum."Quit", "variant"=variant} ("ControlDAQ state cluster"), error in (no error)=w349) -> (error out=w359:errorcluster)  [unwired: 1 in, 2 out]
            n132 = Enqueue Element(queue=w358, element=T21 {"Control storage enum"=enum."Quit", "variant"=variant}, error in (no error)=w359) -> (error out=w356:errorcluster)  [unwired: 1 in, 2 out]
            n133 = Enqueue Element(queue=w355, element=T19 {"Control display enum"=enum."Quit", "variant"=variant}, error in (no error)=w356) -> (error out=w353:errorcluster)  [unwired: 1 in, 2 out]
            n134 = Enqueue Element(queue=w352, element=T17 {"Control Analysis Enum"=enum."Quit", "variant"=variant}, error in (no error)=w353) -> (error out=w346:errorcluster)  [unwired: 1 in, 2 out]
            n135 = Enqueue Element(queue=w345, element=T15 {"Control shutter enum"=enum."Quit", "variant"=variant}, error in (no error)=w346) -> (error out=w343:errorcluster)  [unwired: 1 in, 2 out]
            n136 = call "reset_run_button.vi"("error in"=w343, "Front panel references"=w342) -> ("error out"=w341:errorcluster)  [unwired: 7 in]
            n137 = flat-sequence "Quit event and error handler" {
              tunnel: w341 -> [w364]
              tunnel: [w364] -> w340
              frame #0 {
                n138 = global write "exit.vi" "Exit"(TRUE ("Exit")) -> ()
              }
            }
          }
          frame True {
            n139 = Build Array(cluster{"State Enum":T9, "variant":variant} {"State Enum"=enum."Stop", "variant"=variant} ("element"), cluster{"State Enum":T9, "variant":variant} {"State Enum"=enum."Quit", "variant"=variant} ("element")) -> (w366:cluster{"State Enum":T9, "variant":variant}[])
          }
        }
      }
    }
    "Running" <- w103
    n140 = call "main_state_queue_manager.vi"("error in"=w101, "State array in"=w100, "Main_State_Queue in"=w115) -> ("error out"=w96:errorcluster, "Main_State_Queue out"=w99:refnum<queue>)  [unwired: 7 in]
    n141 = Wait Until Next ms Multiple(millisecond multiple=u32 100) -> ()  [unwired: 1 out]
  }
  n142 = while "Event loop" {
    shift-right: [w373] -> w23
    shift-left: w3 -> [w376]
    tunnel: w34 -> [w377]
    stop <- w374 stop-if-true
    n143 = event shown="[0] \"Quit\": Value Change" {
      selector: _ -> [_ _ _ _ _]
      dyn-events: _ -> [_ _ _ _ _]
      timeout: 0 -> [_ _ _ _ _]
      tunnel: w377 -> [w383 _ w389 w405 w411]
      tunnel: w376 -> [w384 w385 w388 w399 w412]
      tunnel: [w379 w385 w386 w400 w406] -> w373
      tunnel: [TRUE _ _ _ _] -> w375
      event "Quit": Value Change {
        n144 = event-data() -> ()  [unwired: 1 in, 1 out]
        n145 = Enqueue Element(queue=w383, element=cluster{"State Enum":T9, "variant":variant} {"State Enum"=enum."Quit", "variant"=variant}, error in (no error)=w384) -> (error out=w380:errorcluster)  [unwired: 1 in, 2 out]
        n146 = property on="Quit" class="Bool (strict)"(error in=w380, "Value"=FALSE) -> (error out=w379:errorcluster)  [unwired: 1 in, 1 out]
      }
      event Timeout {
        n147 = event-data() -> ()  [unwired: 1 in, 2 out]
      }
      event "Run": Value Change {
        n148 = event-data() -> ()  [unwired: 1 in, 1 out]
        n149 = case shown="True" "Run" {
          tunnel: [cluster{"State Enum":T9, "variant":variant} {"State Enum"=enum."Stop", "variant"=variant} cluster{"State Enum":T9, "variant":variant} {"State Enum"=enum."Start", "variant"=variant}] -> w387
          frame False {
          }
          frame True {
          }
        }
        n150 = Enqueue Element(queue=w389, element=w387, error in (no error)=w388) -> (error out=w386:errorcluster)  [unwired: 1 in, 2 out]
      }
      event Value Change {
        n151 = event-data() -> ()  [unwired: 1 in, 1 out]
        n152 = Bundle(cluster=T7 {"Run mode"=enum."Protocol", "Protocol parameters"={"Repetitions"=0.0, "ON time"=0.0, "OFF time"=0.0, "Stim onset"=0.0, "Stim frequency"=0.0, "Pulse width"=0.0, "Acquire before ON"=0.0, "Acquire after ON"=0.0, "Sync shutter to acquisition"=FALSE}, "Free run parameters"={"Stim onset"=0.0, "Stim frequency"=0.0, "Stim length"=0.0, "Sync shutter to acquisition"=FALSE}, "Device parameters"={"Triggered?"=FALSE, "Shutter channel"="", "Acquisition channels"="", "Acquisition sample rate"=0.0, "Read chunk size"=0, "Stimulation channel"="", "Stimulation sample rate"=0.0}, "Storage parameters"={"Store?"=FALSE, "Path"=path "", "Basename"="", "Auto-increment?"=FALSE}} ("All frontpanel parameters"), "Run mode"="Run mode", "Protocol parameters"="Protocol parameters", "Free run parameters"="Free run parameters", "Device parameters"="Device parameters", "Storage parameters"="Storage parameters") -> (w401:T7)
        n153 = To Variant(anything=w401) -> (Variant=w404:variant)
        n154 = Bundle("State Enum"=main_state_enum."ParamsChanged", "Variant"=w404) -> (w402:cluster{"State Enum":T9, "Variant":variant})  [unwired: 1 in]
        n155 = Enqueue Element(queue=w405, element=w402, error in (no error)=w399) -> (error out=w400:errorcluster)  [unwired: 1 in, 2 out]
      }
      event "Shutter": Value Change {
        n156 = event-data() -> ()  [unwired: 1 in, 1 out]
        n157 = To Variant(anything="Shutter") -> (Variant=w409:variant)
        n158 = Bundle By Name(cluster=cluster{"State Enum":T9, "variant":variant} {"State Enum"=enum."SetShutter", "variant"=variant} ("element"), "variant"=w409) -> (w407:cluster{"State Enum":T9, "variant":variant})
        n159 = Enqueue Element(queue=w411, element=w407, error in (no error)=w412) -> (error out=w406:errorcluster)  [unwired: 1 in, 2 out]
      }
    }
    n160 = global read "exit.vi" "Exit"() -> (w370:bool)
    n161 = Unbundle By Name(w373) -> ("status"=w372:bool)
    n162 = Compound Arithmetic op=OR(w372, w375, w370) -> (w374:bool)
    n163 = Wait Until Next ms Multiple(millisecond multiple=u32 100) -> ()  [unwired: 1 out]
  }
  n164 = Release Queue(queue=w32, error in (no error)=w36) -> (error out=w22:errorcluster)  [unwired: 1 in, 2 out]
  n165 = Merge Errors(w23, w22) -> (w24:errorcluster)
  n166 = call <vilib>:"Simple Error Handler.vi"("type of dialog (OK msg:1)"=w25, "error in (no error)"=w24) -> ()  [unwired: 3 in, 5 out]
